vi "Configure Waveform (Voltage).vi"(6 "Settle (1mS)":u32=1, 7 "Step & Counter":cluster{"Step (0: Once)":u16, "Counter (1)":i32}={"Step (0: Once)"=0, "Counter (1)"=1} {"Counter (1)" min=1 max=9999 step=1; "Step (0: Once)" items=["Once", "Auto"]}, 8 "error in (no error)":errorcluster, 9 "Time Points":dbl[](array[numeric]) format="%#_6f", 10 "Value Points":dbl[](array[numeric]) format="%#_6f", 11 "VISA resource name":refnum<visa-resource-name>) -> (0 "error out":errorcluster, 3 "VISA resource name out":refnum<visa-resource-name>)   [LabVIEW 2012, in "TDK-Lambda Z.lvlib"]
doc: "Configures WAVE -This mode occurs when the VOLT:MODE WAVE command is programmed. \n In this mode of output operation, the triggered output voltage and rise and fall slope are specified within a list and the trigger controls the sequencing through the values in the list."
uses:
  TDK-Lambda Z.lvlib
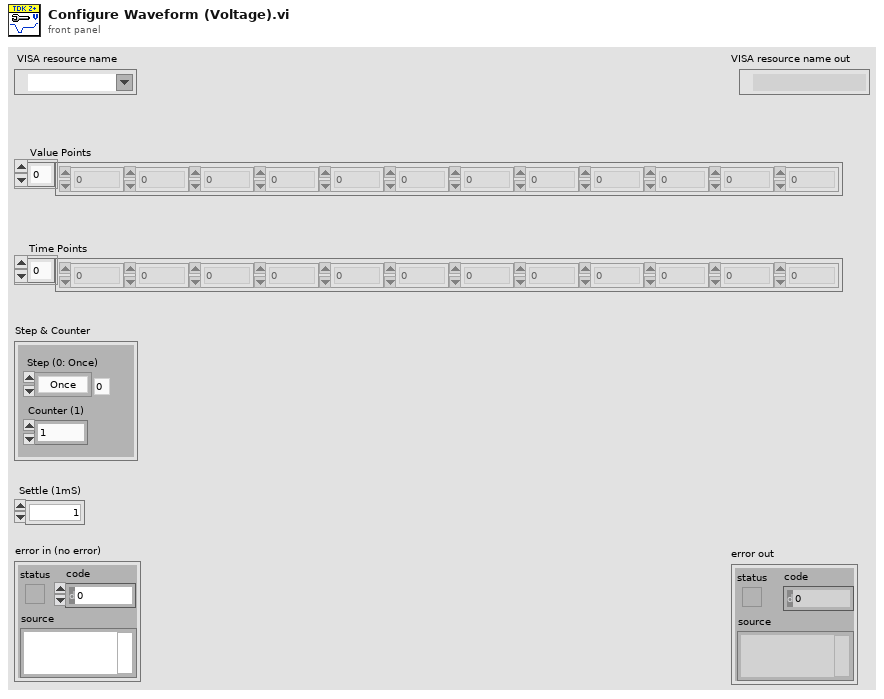
[diagram p1: front panel]
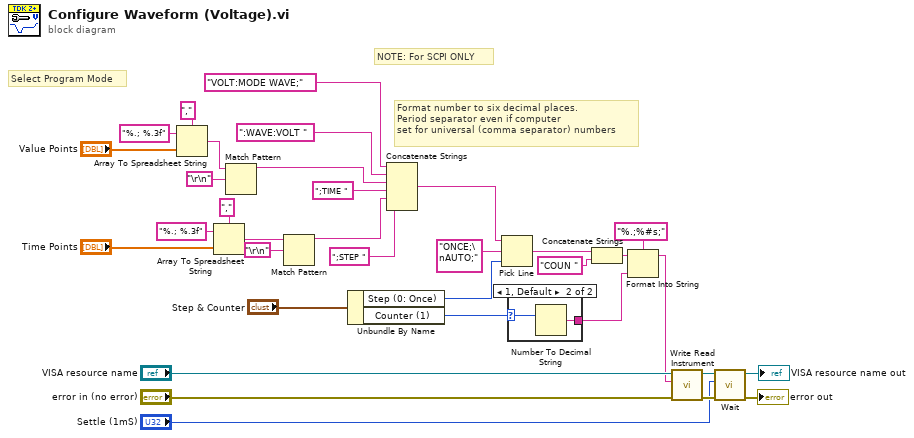
[diagram p0: block diagram]
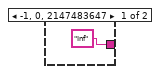
[diagram p2: hidden frame]
diagram:
  # "Select Program Mode"
  # "NOTE: For SCPI ONLY"
  # "Format number to six decimal places.\nPeriod separator even if computer \nset for universal (comma separator) numbers"
  n1 = Array To Spreadsheet String(delimiter (Tab)=",", array="Value Points", 3:"%.; %.3f" ("format string")) -> (spreadsheet string=w18:string)
  n2 = Array To Spreadsheet String(delimiter (Tab)=",", array="Time Points", 3:"%.; %.3f" ("format string")) -> (spreadsheet string=w15:string)
  n3 = Match Pattern(string=w18, regular expression="\r\n") -> (before substring=w1:string)  [unwired: 1 in, 3 out]
  n4 = Match Pattern(string=w15, regular expression="\r\n") -> (before substring=w6:string)  [unwired: 1 in, 3 out]
  n5 = Unbundle By Name("Step & Counter") -> ("Step (0: Once)"=w25:u16, "Counter (1)"=w24:i32)
  n6 = Concatenate Strings("VOLT:MODE WAVE;" ("concatenated string"), ":WAVE:VOLT " ("string"), w1, ";TIME " ("string"), w6, ";STEP " ("string")) -> (w5:string)
  n7 = Pick Line(string ("")=w5, multi-line string="ONCE;\nAUTO;" ("format string"), line index=w25) -> (output string=w10:string)
  n8 = case shown="1, Default" w24 {
    selector: w24 -> [_ w37]
    tunnel: ["Inf" w36] -> w23
    frame -1, 0, 2147483647 {
    }
    frame 1, Default {
      n9 = Number To Decimal String(number=w37) -> (decimal integer string=w36:string)  [unwired: 1 in]
    }
  }
  n10 = Concatenate Strings(w10, "COUN " ("string")) -> (w7:string)
  n11 = Format Into String(format string="%.;%#s;", initial string=w7, w23) -> (resulting string=w27:string)  [unwired: 1 in, 1 out]
  n12 = call "Write Read Instrument.vi"("error in (no error)"="error in (no error)", "SCPI  Write Command/Query"=w27, "VISA resource name"="VISA resource name") -> ("error out"=w31:errorcluster, "VISA resource name out"=w32:refnum<visa-resource-name>)  [unwired: 6 in, 1 out]
  n13 = call "Wait.vi"("error in (no error)"=w31, "Wait (1mS)"="Settle (1mS)", "VISA resource name"=w32) -> ("error out"=→"error out":errorcluster, "VISA resource name out"=→"VISA resource name out":refnum<visa-resource-name>)  [unwired: 7 in]
